vi "update.vi"(8 "error in (no error)":errorcluster, 10 "update":refnum<class "GenericImageProcessor.lvclass">, 11 "GenericImageProcessor in":refnum<class "GenericImageProcessor.lvclass">) -> (0 "error out":errorcluster, 3 "GenericImageProcessor out":refnum<class "GenericImageProcessor.lvclass">)   [LabVIEW 2010, in "GenericImageProcessor.lvclass"]
uses:
  GenericImageProcessor.lvclass
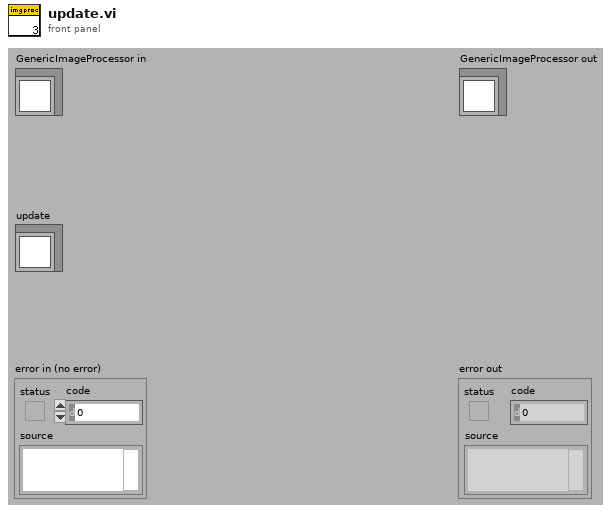
[diagram p1: front panel]
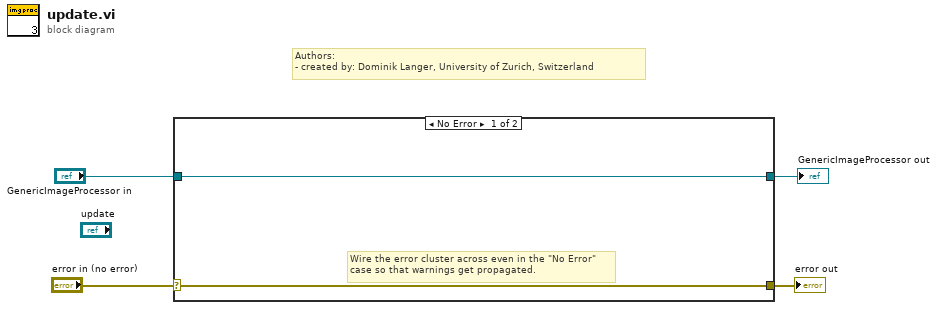
[diagram p0: block diagram]
diagram:
  # "Authors: \n- created by: Dominik Langer, University of Zurich, Switzerland"
  n1 = case shown="No Error" "error in (no error)" {
    selector: "error in (no error)" -> [w5 w8]
    tunnel: [w5 w8] -> w3
    tunnel: [w6 w7] -> w1
    tunnel: "GenericImageProcessor in" -> [w6 w7]
    frame No Error {
      # "Wire the error cluster across even in the \"No Error\"\ncase so that warnings get propagated."
    }
    frame Error {
    }
  }
  "error out" <- w3
  "GenericImageProcessor out" <- w1
